vi "MergeCells.vi"(8 "error":errorcluster caption="错误输入（无错误）", 9 "Second Cell":string, 10 "First Cell":string, 11 "Excel._Worksheet":refnum<k7>) -> (0 "error out":errorcluster caption="错误输出", 3 "Excel._Worksheet":refnum<k7>)   [LabVIEW 2009]
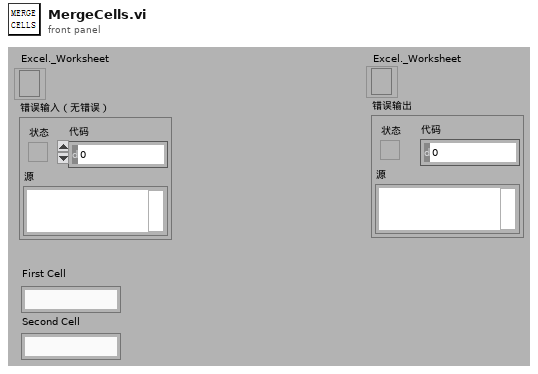
[diagram p1: front panel]
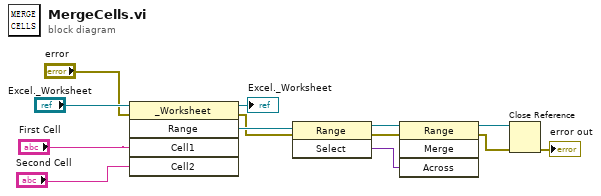
[diagram p0: block diagram]
diagram:
  n1 = invoke class="_Worksheet" method="Range"(reference="Excel._Worksheet", error in="error", "Cell1"="First Cell", "Cell2"="Second Cell") -> (reference out=→"Excel._Worksheet":refnum<k7>, error out=w7:errorcluster, "Range"=w11:refnum<k7>)  [unwired: 1 in, 2 out]
  n2 = invoke class="Range" method="Select"(reference=w11, error in=w7) -> (reference out=w2:refnum<k7>, error out=w8:errorcluster, "Select"=w1:variant)  [unwired: 1 in]
  n3 = invoke class="Range" method="Merge"(reference=w2, error in=w8, "Across"=w1) -> (reference out=w10:refnum<k7>, error out=w9:errorcluster)  [unwired: 1 in, 2 out]
  n4 = Close Reference(reference=w10, error in (no error)=w9) -> (error out=→"error out":errorcluster)
